vi "Get Value by Array (String Value).vi"(8 "error in (no error)":errorcluster, 10 "Keys":string[](array[string]), 11 "JSON Value in":refnum<class "JSON Value.lvclass">) -> (0 "error out":errorcluster, 2 "value":string)   [LabVIEW 2016, in "JSON Value.lvclass"]
uses:
  JSON Value.lvclass
  Get Value by Array (JSON).vi
  Read Value/Read value as String.vi
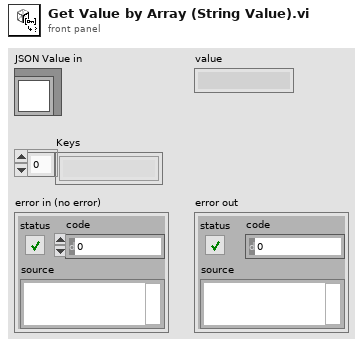
[diagram p1: front panel]
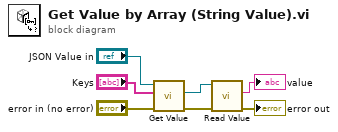
[diagram p0: block diagram]
diagram:
  n1 = call-poly "Get Value.vi"("error in (no error)"="error in (no error)", "Keys"="Keys", "JSON Value in"="JSON Value in") -> ("error out"=w1:errorcluster, "JSON Value out"=w2:refnum<class "JSON Value.lvclass">)  [unwired: 7 in]
  n2 = call-poly "Read Value.vi"("error in (no error)"=w1, "JSON String in"=w2) -> ("error out"=→"error out":errorcluster, "value"=→"value":string)  [unwired: 8 in]
